vi "Calculate_Absolute_distance.vi"(8 "Error In":errorcluster, 10 "data in":string, 11 "Refnum In":refnum<vi>) -> (0 "Error Out":errorcluster, 1 "Prepart contact in mm":dbl, 2 "Absolute distance in inch":dbl, 3 "Refnum out":refnum<vi>, 4 "Prepart contact in inch":dbl, 5 "Absolute distance in mm":dbl)   [LabVIEW 2017]
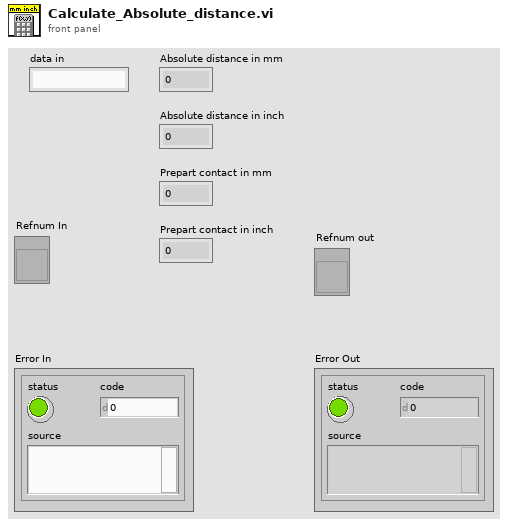
[diagram p1: front panel]
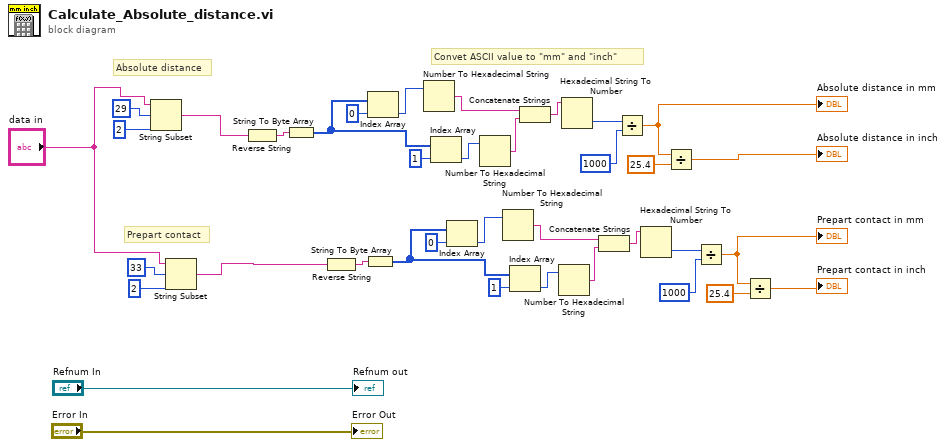
[diagram p0: block diagram]
diagram:
  # "Convet ASCII value to \"mm\" and \"inch\""
  # "Prepart contact"
  # "Absolute distance"
  n1 = String Subset(string="data in", offset (0)=29, length (rest)=2 ("length (rest)")) -> (substring=w5:string)
  n2 = String Subset(string="data in", offset (0)=33, length (rest)=2 ("length (rest)")) -> (substring=w37:string)
  n3 = Reverse String(1:w5) -> (0:w6:string)
  n4 = String To Byte Array(string=w6) -> (unsigned byte array=w11:u8[])
  n5 = Reverse String(1:w37) -> (0:w36:string)
  n6 = String To Byte Array(string=w36) -> (unsigned byte array=w31:u8[])
  n7 = Index Array(array=w11, index=0) -> (element=w8:u8)
  n8 = Number To Hexadecimal String(2:w8) -> (0:w13:string)  [unwired: 1 in]
  n9 = Index Array(array=w11, index=1) -> (element=w9:u8)
  n10 = Index Array(array=w31, index=0) -> (element=w34:u8)
  n11 = Number To Hexadecimal String(2:w9) -> (0:w12:string)  [unwired: 1 in]
  n12 = Number To Hexadecimal String(2:w34) -> (0:w29:string)  [unwired: 1 in]
  n13 = Index Array(array=w31, index=1) -> (element=w33:u8)
  n14 = Concatenate Strings(w13, w12) -> (w14:string)
  n15 = Number To Hexadecimal String(2:w33) -> (0:w30:string)  [unwired: 1 in]
  n16 = Hexadecimal String To Number(string=w14) -> (number=w15:u32)  [unwired: 2 in, 1 out]
  n17 = Concatenate Strings(w29, w30) -> (w28:string)
  n18 = Divide(x=w15, y=1000) -> (x/y=w17:dbl)
  "Absolute distance in mm" <- w17
  n19 = Hexadecimal String To Number(string=w28) -> (number=w27:u32)  [unwired: 2 in, 1 out]
  n20 = Divide(x=w17, y=25.4) -> (x/y=→"Absolute distance in inch":dbl)
  n21 = Divide(x=w27, y=1000) -> (x/y=w25:dbl)
  "Prepart contact in mm" <- w25
  n22 = Divide(x=w25, y=25.4) -> (x/y=→"Prepart contact in inch":dbl)
  "Error Out" <- "Error In"
  "Refnum out" <- "Refnum In"
